vi "Clicked.vi"(0 "reference in":refnum<class "Button.lvclass">, 5 "error in (no error)":errorcluster) -> (14 "reference out":refnum<class "Button.lvclass">, 15 "Array":string[](array[string]), 19 "error out":errorcluster)   [LabVIEW 2019, in "Button.lvclass"]
uses:
  Button.lvclass
  C:/Users/Taylor.Hillegeist/OneDrive - Ultra/LabVIEW/Pgui2/Pgui_Obj_class/Pgui_Obj.lvclass
  Pgui_Obj_class/Pgui_Obj.lvclass
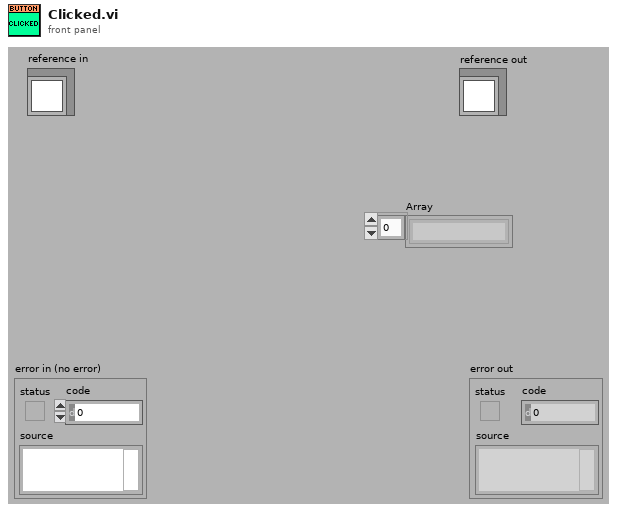
[diagram p1: front panel]
types:
  T1 = typedef "Button.lvclass/ObjectAttributes.ctl" = cluster{"Text":string, "Override size":cluster{"Width":i16, "Height":i16}}
  T2 = typedef "Pgui_Obj.lvclass/ObjectAttributes.ctl" = cluster{"Children":refnum<class "Pgui_Obj.lvclass">[], "Draw Instr":picture, "Params":cluster{"left":i16, "top":i16, "right":i16, "bottom":i16}, "Parent_Pgui_Obj":refnum<class "Pgui_Obj.lvclass">, "MouseOver":bool}
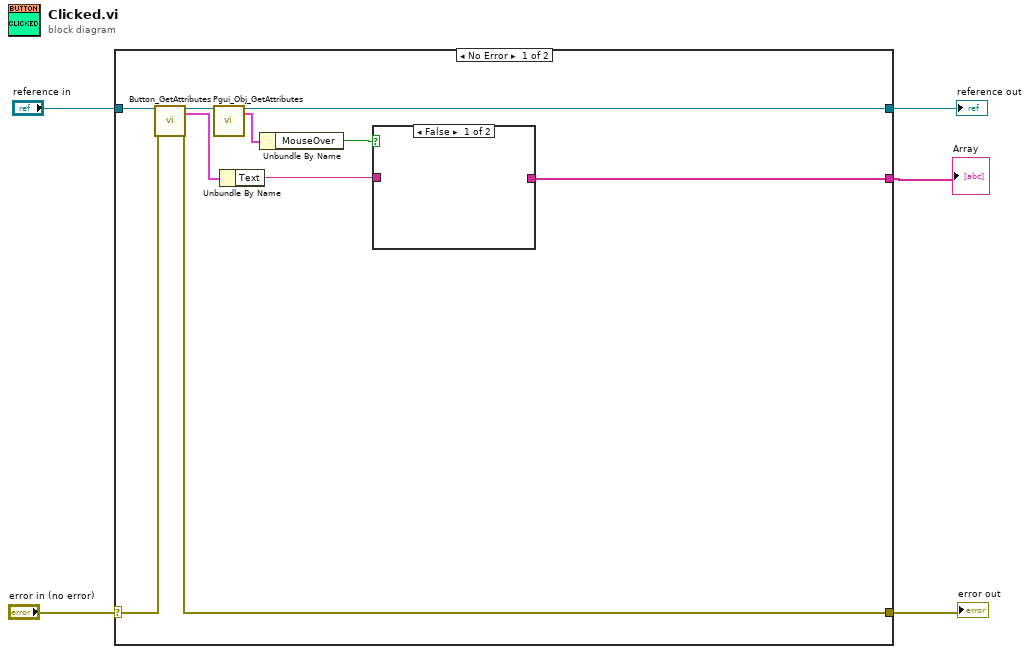
[diagram p0: block diagram]
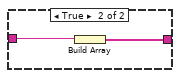
[diagram p2: hidden frame]
diagram:
  n1 = case shown="No Error" "error in (no error)" {
    selector: "error in (no error)" -> [w15 w19]
    tunnel: [w13 w19] -> w4
    tunnel: [w10 w18] -> w2
    tunnel: "reference in" -> [w12 w18]
    tunnel: [w7 _] -> w1
    frame No Error {
      n2 = call "Button_GetAttributes.vi"("reference in"=w12, "error in (no error)"=w15) -> ("reference out"=w11:refnum<class "Button.lvclass">, "Data"=w14:T1, "error out"=w13:errorcluster)  [unwired: 14 in, 1 out]
      n3 = call "Pgui_Obj_GetAttributes.vi"("reference in"=w11) -> ("reference out"=w10:refnum<class "Button.lvclass">, "Data"=w9:T2)  [unwired: 15 in, 2 out]
      n4 = Unbundle By Name(w14) -> ("Text"=w8:string)
      n5 = Unbundle By Name(w9) -> ("MouseOver"=w6:bool)
      n6 = case shown="False" w6 {
        tunnel: w8 -> [_ w17]
        tunnel: [_ w16] -> w7
        frame False {
        }
        frame True {
          n7 = Build Array(w17) -> (w16:string[])
        }
      }
    }
    frame Error {
    }
  }
  "error out" <- w4
  "reference out" <- w2
  "Array" <- w1
